vi "U01_8_3 CloseExcelActiveX.vi"(6 "Save?":bool, 8 "error in (no error)":errorcluster, 11 "References":T1) -> (0 "error out":errorcluster)   [LabVIEW 2019]
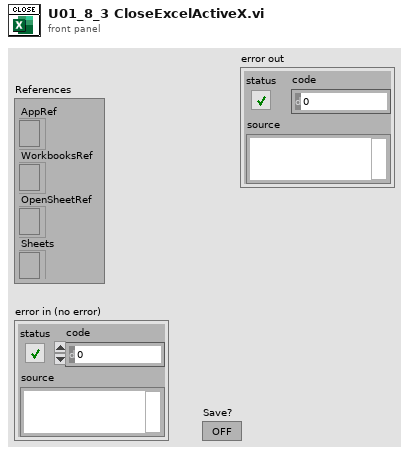
[diagram p1: front panel]
types:
  T1 = cluster{"AppRef":refnum<k7>, "WorkbooksRef":refnum<k7>, "OpenSheetRef":refnum<k7>, "Sheets":refnum<k7>}
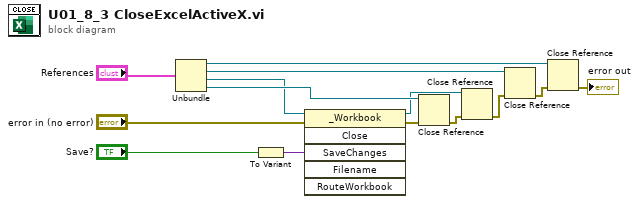
[diagram p0: block diagram]
diagram:
  n1 = Unbundle("References") -> ("AppRef"=w11:refnum<k7>, "WorkbooksRef"=w12:refnum<k7>, "OpenSheetRef"=w13:refnum<k7>, "Sheets"=w14:refnum<k7>)
  n2 = To Variant(anything="Save?") -> (Variant=w3:variant)
  n3 = invoke class="_Workbook" method="Close"(reference=w13, error in="error in (no error)", "SaveChanges"=w3) -> (reference out=w7:refnum<k7>, error out=w5:errorcluster)  [unwired: 3 in, 4 out]
  n4 = Close Reference(reference=w14, error in (no error)=w5) -> (error out=w6:errorcluster)
  n5 = Close Reference(reference=w7, error in (no error)=w6) -> (error out=w8:errorcluster)
  n6 = Close Reference(reference=w12, error in (no error)=w8) -> (error out=w9:errorcluster)
  n7 = Close Reference(reference=w11, error in (no error)=w9) -> (error out=→"error out":errorcluster)
